vi "DMA Pause Global.vi"(0 "Pause IN":bool, 5 "Error IN":errorcluster, 8 "Mode":T1) -> (14 "Pause":bool[](array[boolean]), 19 "Error OUT":errorcluster)   [LabVIEW 2019]
uses:
  Type Defs/Crash File Mode.ctl
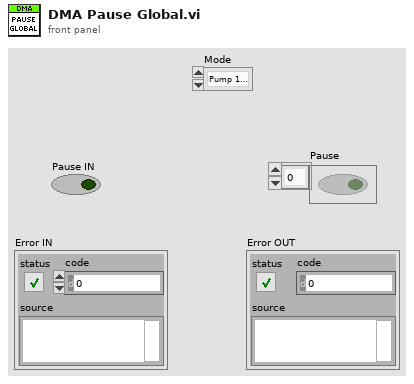
[diagram p1: front panel]
types:
  T1 = typedef "Crash File Mode.ctl" = enum16{"Pump 1 Write", "Pump 2 Write", "Pump 3 Write", "Pump 4 Write", "Pump 5 Write", "Pump 6 Write", "Read All", "Init"}
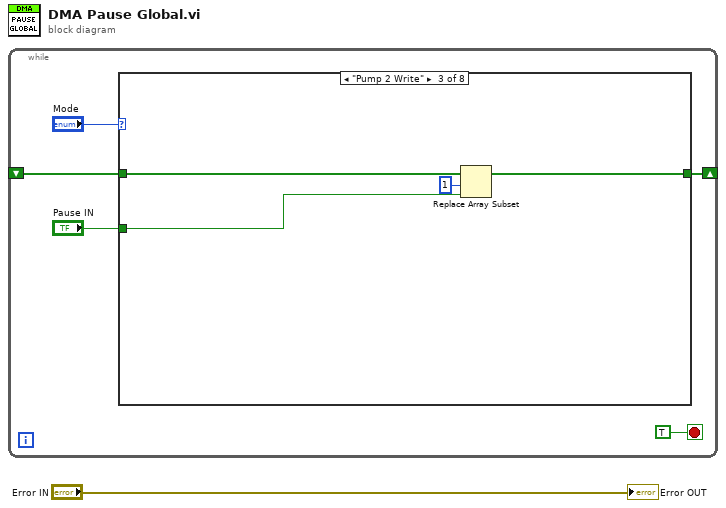
[diagram p0: block diagram]
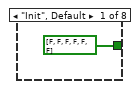
[diagram p2: hidden frame]
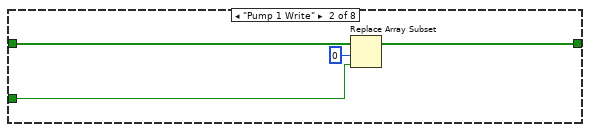
[diagram p3: hidden frame]
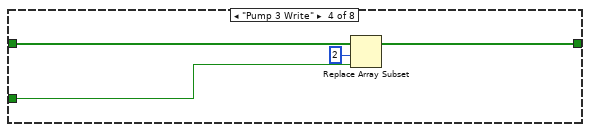
[diagram p4: hidden frame]
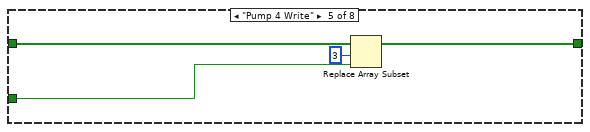
[diagram p5: hidden frame]
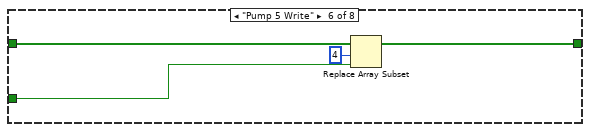
[diagram p6: hidden frame]
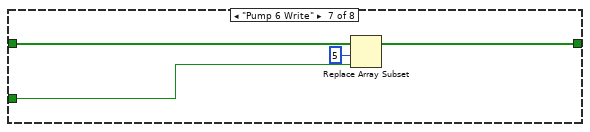
[diagram p7: hidden frame]
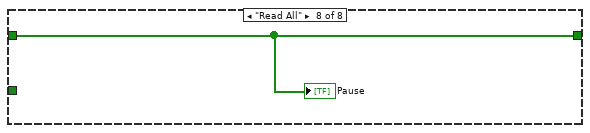
[diagram p8: hidden frame]
diagram:
  n1 = while {
    shift-right: [w4] -> _
    shift-left: _ -> [w3]
    stop <- TRUE stop-if-true
    n2 = case shown="\"Pump 2 Write\"" "Mode" {
      tunnel: [bool[] [FALSE, FALSE, FALSE, FALSE, FALSE, FALSE] w10 w14 w18 w22 w26 w30 w32] -> w4
      tunnel: w3 -> [_ w11 w15 w19 w23 w27 w31 w32]
      tunnel: "Pause IN" -> [_ w8 w12 w16 w20 w24 w28 _]
      frame "Init", Default {
      }
      frame "Pump 1 Write" {
        n3 = Replace Array Subset(array=w11, new element=w8, index=0) -> (w10:bool[])
      }
      frame "Pump 2 Write" {
        n4 = Replace Array Subset(array=w15, new element=w12, index=1) -> (w14:bool[])
      }
      frame "Pump 3 Write" {
        n5 = Replace Array Subset(array=w19, new element=w16, index=2) -> (w18:bool[])
      }
      frame "Pump 4 Write" {
        n6 = Replace Array Subset(array=w23, new element=w20, index=3) -> (w22:bool[])
      }
      frame "Pump 5 Write" {
        n7 = Replace Array Subset(array=w27, new element=w24, index=4) -> (w26:bool[])
      }
      frame "Pump 6 Write" {
        n8 = Replace Array Subset(array=w31, new element=w28, index=5) -> (w30:bool[])
      }
      frame "Read All" {
        "Pause" <- w32
      }
    }
  }
  "Error OUT" <- "Error IN"
